vi "Filter vi if in vi lib or others.vi"(4 "error in":errorcluster, 5 "Include .ctl's":bool, 6 "Include .vi's":bool=TRUE, 7 "vi reference in":refnum<vi>) -> (0 "error out":errorcluster, 1 "Boolean":bool, 2 "Path":path, 3 "vi reference (dup)":refnum<vi>)   [LabVIEW 2010]
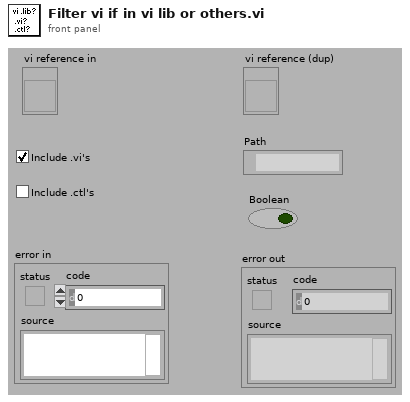
[diagram p1: front panel]
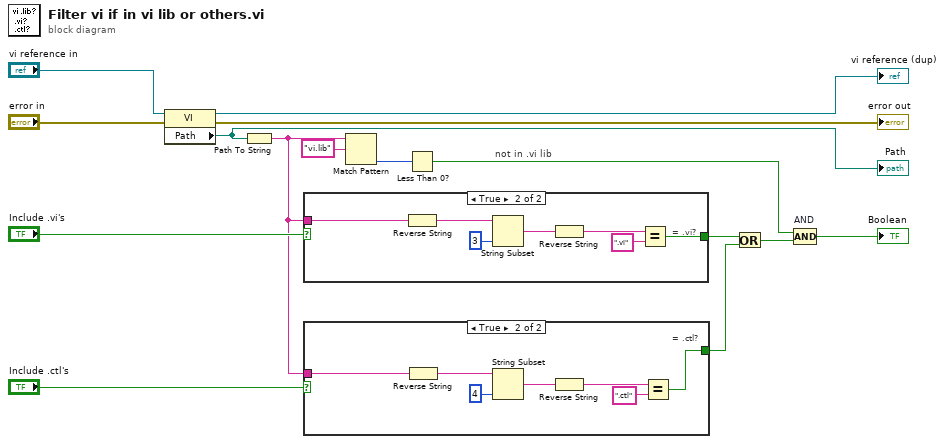
[diagram p0: block diagram]
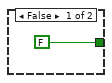
[diagram p2: hidden frame]
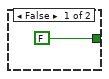
[diagram p3: hidden frame]
diagram:
  # "not in .vi lib"
  n1 = property class="VI"(reference="vi reference in", error in="error in") -> (reference out=→"vi reference (dup)":refnum<vi>, error out=→"error out":errorcluster, "Path"=w11:path)
  "Path" <- w11
  n2 = Path To String(path=w11) -> (string=w4:string)
  n3 = case shown="True" "Include .vi's" {
    tunnel: w4 -> [_ w18]
    tunnel: [FALSE w17] -> w6
    frame False {
    }
    frame True {
      # "= .vi?"
      n4 = Reverse String(1:w18) -> (0:w23:string)
      n5 = String Subset(string=w23, length (rest)=3 ("length (rest)")) -> (substring=w21:string)  [unwired: 1 out]
      n6 = Reverse String(1:w21) -> (0:w20:string)
      n7 = Equal?(x=w20, y=".vi") -> (x = y?=w17:bool)
    }
  }
  n8 = case shown="True" "Include .ctl's" {
    tunnel: w4 -> [_ w26]
    tunnel: [FALSE w25] -> w7
    frame False {
    }
    frame True {
      # "= .ctl?"
      n9 = Reverse String(1:w26) -> (0:w27:string)
      n10 = String Subset(string=w27, length (rest)=4 ("length (rest)")) -> (substring=w29:string)  [unwired: 1 out]
      n11 = Reverse String(1:w29) -> (0:w30:string)
      n12 = Equal?(x=w30, y=".ctl") -> (x = y?=w25:bool)
    }
  }
  n13 = Match Pattern(string=w4, regular expression="vi.lib") -> (offset past match=w5:i32)  [unwired: 4 out]
  n14 = Less Than 0?(x=w5) -> (x < 0?=w8:bool)
  n15 = Or(x=w6, y=w7) -> (x .or. y?=w9:bool)
  n16 = Compound Arithmetic op=AND "AND"(w8, w9) -> (→"Boolean":bool)
